vi "Create CCD Camera Class.vi"(8 "error in (no error)":errorcluster, 11 "Channel in":refnum<class "Channel.lvclass">) -> (0 "error out":errorcluster, 3 "Channel out":refnum<class "Channel.lvclass">)   [LabVIEW 2018, in "Channel.lvclass"]
uses:
  Channel.lvclass
  Simulated_Image_Constructor/Simulated_Image_Constructor.lvclass
  Image Constructor/Image Constructor.lvclass
  C:/Users/observer/Desktop/SPARC4_ACS/Simulated_Image_Constructor/Simulated_Image_Constructor.lvclass
  CCDCamera/CCDCamera.lvclass
  C:/Users/observer/Desktop/SPARC4_ACS/Simulated_CCD_Camera/Simulated_CCD_Camera.lvclass
  Cooler/Cooler.lvclass
  C:/Users/observer/Desktop/SPARC4_ACS/Simulated_Cooler/Simulated_Cooler.lvclass
  Header/Header.lvclass
  C:/Users/observer/Desktop/SPARC4_ACS/Simulated_Header/Simulated_Header.lvclass
  Simulated_Image_Constructor/Simulated_Image_Constructor.lvclass/Simulated_Image_Constructor.ctl
  Channel.lvclass/Channel.ctl
  Save Image/Save Image.lvclass
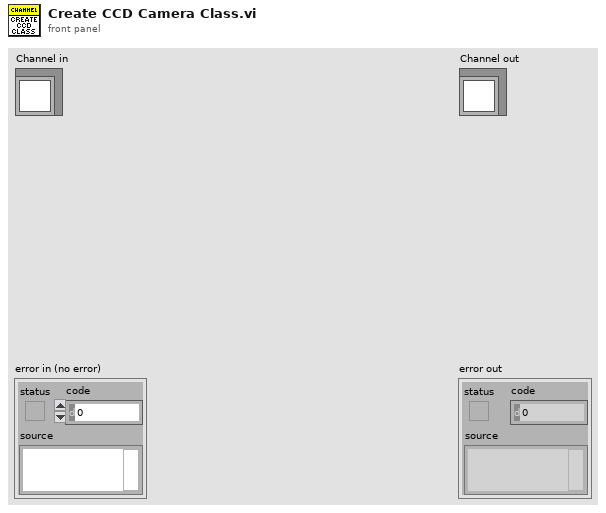
[diagram p1: front panel]
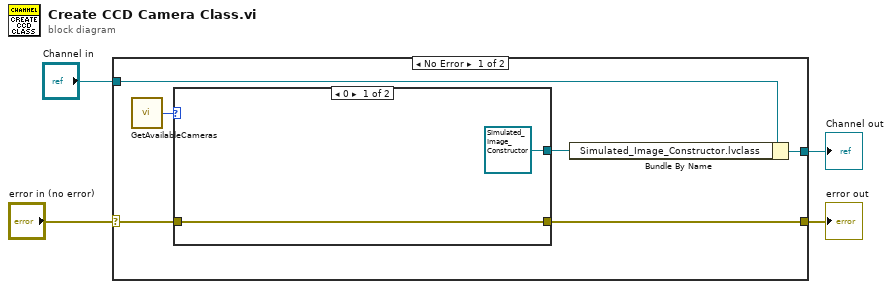
[diagram p0: block diagram]
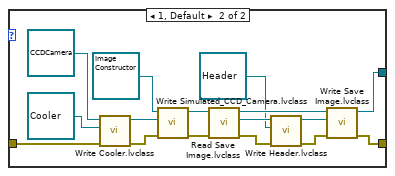
[diagram p2: hidden frame]
diagram:
  n1 = case shown="No Error" "error in (no error)" {
    selector: "error in (no error)" -> [w7 w30]
    tunnel: [w5 w30] -> w3
    tunnel: [w10 w29] -> w1
    tunnel: "Channel in" -> [w9 w29]
    frame No Error {
      n2 = call <userlib>:"GetAvailableCameras.vi"() -> ("totalCameras"=w8:i32)  [unwired: 3 in, 2 out]
      n3 = case shown="0" w8 {
        tunnel: w7 -> [w12 w25]
        tunnel: [refnum<class "Simulated_Image_Constructor.lvclass"> refnum ("Simulated_Image_Constructor.lvclass") w14] -> w6
        tunnel: [w12 w13] -> w5
        frame 0 {
        }
        frame 1, Default {
          n4 = call-dynamic "Write Cooler.lvclass.vi"("error in (no error)"=w25, "Simulated_Cooler.lvclass"=refnum<class "Cooler.lvclass"> refnum ("Cooler.lvclass"), "CCDCamera in"=refnum<class "CCDCamera.lvclass"> refnum ("CCDCamera.lvclass")) -> ("error out"=w23:errorcluster, "CCDCamera out"=w24:refnum<class "CCDCamera.lvclass">)  [unwired: 7 in]
          n5 = call "Write Simulated_CCD_Camera.lvclass.vi"("error in (no error)"=w23, "Simulated_CCD_Camera.lvclass"=w24, "Image Constructor in"=refnum<class "Image Constructor.lvclass"> refnum ("Image Constructor.lvclass")) -> ("error out"=w21:errorcluster, "Image Constructor out"=w22:refnum<class "Image Constructor.lvclass">)  [unwired: 7 in]
          n6 = call "Read Save Image.lvclass.vi"("error in (no error)"=w21, "Image Constructor in"=w22) -> ("error out"=w17:errorcluster, "Save Image.lvclass"=w19:refnum<class "Save Image.lvclass">, "Image Constructor out"=w20:refnum<class "Image Constructor.lvclass">)  [unwired: 7 in]
          n7 = call "Write Header.lvclass.vi"("error in (no error)"=w17, "Simulated_Header.lvclass"=refnum<class "Header.lvclass"> refnum ("Header.lvclass"), "Save Image in"=w19) -> ("error out"=w16:errorcluster, "Save Image out"=w18:refnum<class "Save Image.lvclass">)  [unwired: 7 in]
          n8 = call "Write Save Image.lvclass.vi"("error in (no error)"=w16, "Save Image.lvclass"=w18, "Image Constructor in"=w20) -> ("error out"=w13:errorcluster, "Image Constructor out"=w14:refnum<class "Image Constructor.lvclass">)  [unwired: 7 in]
        }
      }
      n9 = Bundle By Name(cluster=w9, "Simulated_Image_Constructor.lvclass"=w6) -> (w10:refnum<class "Channel.lvclass">)
    }
    frame Error {
    }
  }
  "error out" <- w3
  "Channel out" <- w1
